vi "Configure Dialog.vi"(8 "Error In":errorcluster, 11 "Mute Single Msg in":refnum<class "Mute Single Msg.lvclass">) -> (0 "Error Out":errorcluster, 2 "OK?":bool, 3 "Mute Single Msg out":refnum<class "Mute Single Msg.lvclass">)   [LabVIEW 2016, in "KIT-QVA.lvlib" / "Mute Single Msg.lvclass"]
doc: "This overrides of this dynamic dispatch VI open the frontpanel to set derived message attributes."
uses:
  Mute Single Msg.lvclass
  Mute Single Msg.lvclass/Mute Single Msg.ctl
panel:
  in  "Detector":u8
  in  "Mute":bool
  in  "OK":bool
  in  "Cancel":bool
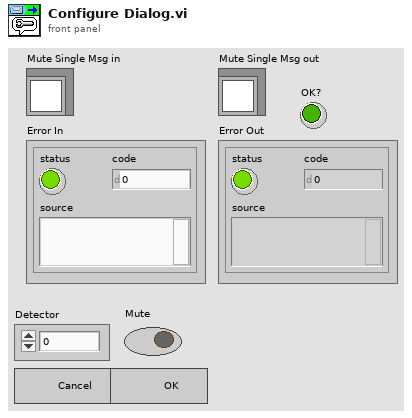
[diagram p1: front panel]
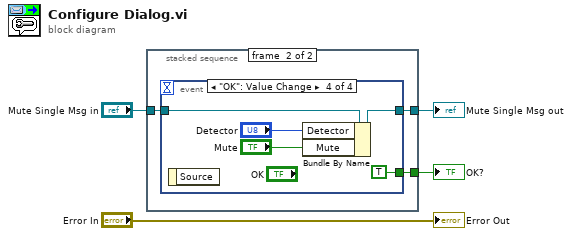
[diagram p0: block diagram]
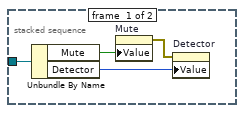
[diagram p2: hidden frame]
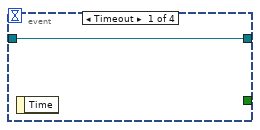
[diagram p3: hidden frame]
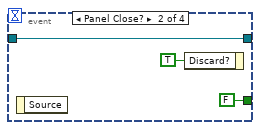
[diagram p4: hidden frame]
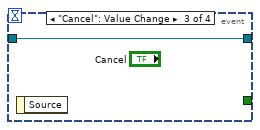
[diagram p5: hidden frame]
diagram:
  n1 = stacked-sequence {
    tunnel: "Mute Single Msg in" -> [w8 w11]
    tunnel: [_ w10] -> w2
    tunnel: [_ w9] -> w1
    frame #0 {
      n2 = Unbundle By Name(w8) -> ("Mute"=w7:bool, "Detector"=w6:u8)
      n3 = property on="Mute" class="Bool (strict)"("Value"=w7) -> (error out=w5:errorcluster)  [unwired: 2 in, 1 out]
      n4 = property on="Detector" class="DigNum (strict)"(error in=w5, "Value"=w6) -> ()  [unwired: 1 in, 2 out]
    }
    frame #1 {
      n5 = event shown="[3] \"OK\": Value Change" {
        selector: _ -> [_ _ _ _]
        dyn-events: _ -> [_ _ _ _]
        timeout: _ -> [_ _ _ _]
        tunnel: [w12 w13 w16 w20] -> w10
        tunnel: w11 -> [w12 w13 w16 w21]
        tunnel: [_ FALSE _ TRUE] -> w9
        event Timeout {
          n6 = event-data() -> ()  [unwired: 1 in, 1 out]
        }
        event Panel Close? {
          n7 = event-data() -> ()  [unwired: 1 in, 1 out]
          n8 = event-data("Discard?"=TRUE) -> ()  [unwired: 1 in, 1 out]
        }
        event "Cancel": Value Change {
          n9 = event-data() -> ()  [unwired: 1 in, 1 out]
        }
        event "OK": Value Change {
          n10 = event-data() -> ()  [unwired: 1 in, 1 out]
          n11 = Bundle By Name(cluster=w21, "Detector"="Detector", "Mute"="Mute") -> (w20:refnum<class "Mute Single Msg.lvclass">)
        }
      }
    }
  }
  "Mute Single Msg out" <- w2
  "OK?" <- w1
  "Error Out" <- "Error In"
